vi "Load General Challenge Config Data.vi"(8 "Error In":errorcluster, 9 "Challenge Directory":path, 10 "Challenge Config":T1, 11 "Config File Handle":T2) -> (0 "Error Out":errorcluster, 1 "Challenge Directory":path, 2 "Challenge Config":T1, 3 "Config File Handle":T2)   [LabVIEW 2013, in "VIChallenge.lvlib"]
doc: "This VI loads the general challenge config data from the challenge ini"
uses:
  VIChallenge.lvlib
  <vilib>/Utility/config.llb/Config Data RefNum.ctl
  Type Defs/Challenge.ctl
  <vilib>/Utility/config.llb/Read Key (I32).vi
  <vilib>/Utility/config.llb/Read Key (String).vi
  <vilib>/Utility/config.llb/NI_LVConfig.lvlib
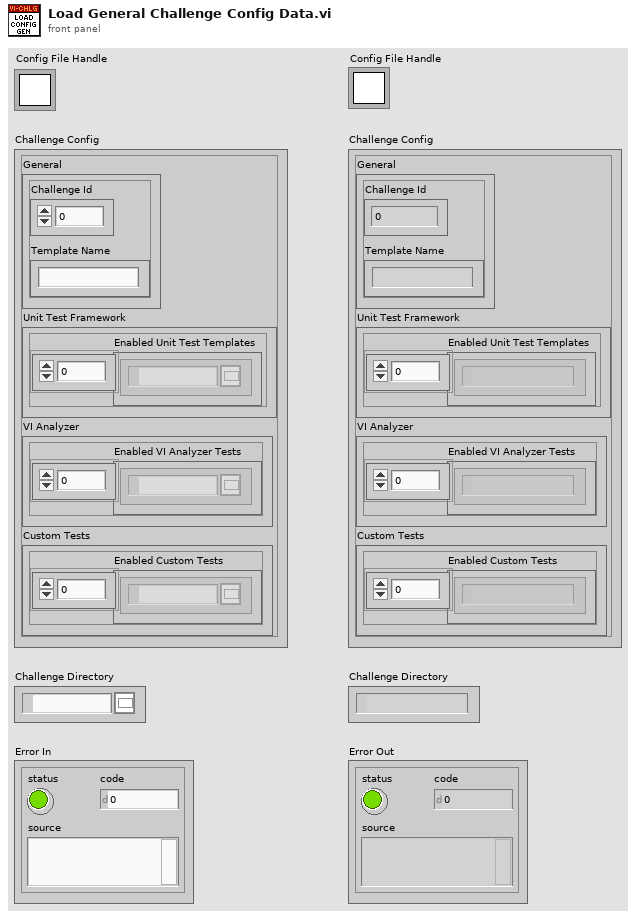
[diagram p1: front panel]
types:
  T1 = typedef "VIChallenge.lvlib/Challenge.ctl" = cluster{"General":cluster{"Challenge Id":i32, "Template Name":string}, "Unit Test Framework":cluster{"Enabled Unit Test Templates":path[]}, "VI Analyzer":cluster{"Enabled VI Analyzer Tests":path[]}, "Custom Tests":cluster{"Enabled Custom Tests":path[]}}
  T2 = typedef "NI_LVConfig.lvlib/Config Data RefNum.ctl" = refnum<k1>
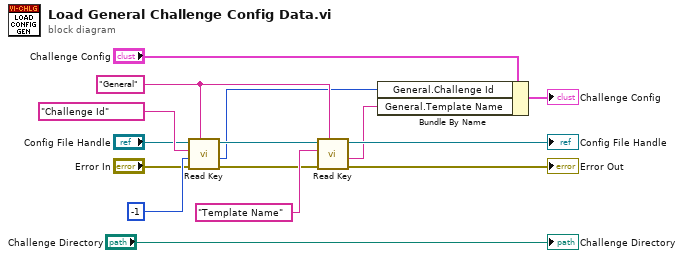
[diagram p0: block diagram]
diagram:
  w14 = "General" ("section")
  n1 = call-poly <vilib>:"Read Key.vi"("section"=w14, "error in (no error)"="Error In", "default value"=-1, "key"="Challenge Id", "refnum"="Config File Handle") -> ("error out"=w13:errorcluster, "value"=w5:i32, "refnum out"=w12:T2)  [unwired: 3 in, 1 out]
  n2 = call-poly <vilib>:"Read Key.vi"("section"=w14, "error in (no error)"=w13, "key"="Template Name", "refnum"=w12) -> ("error out"=→"Error Out":errorcluster, "value"=w4:string, "refnum out"=→"Config File Handle":T2)  [unwired: 4 in, 1 out]
  n3 = Bundle By Name(cluster="Challenge Config", "General.Challenge Id"=w5, "General.Template Name"=w4) -> (→"Challenge Config":T1)
  "Challenge Directory" <- "Challenge Directory"
